vi "Replace Missing Denpendency VIs - Custom gRPC Service Core.vi"(8 "error in":errorcluster, 10 "gRPC Service Name":string, 11 "VI Refnum":refnum<vi>) -> (0 "error out":errorcluster)   [LabVIEW 2023, in "Plugin Generator.lvlib"]
uses:
  Plugin Generator.lvlib
  <vilib>/Utility/traverseref.llb/TRef TravTarget.ctl
  <vilib>/Utility/traverseref.llb/VI Scripting - Traverse.lvlib
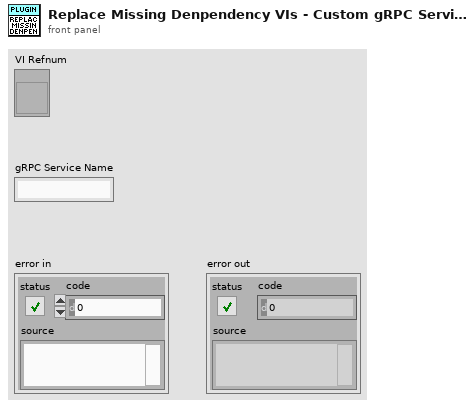
[diagram p1: front panel]
types:
  T1 = typedef "TRef TravTarget.ctl" = enum16{"FP", "BD", "Other"}
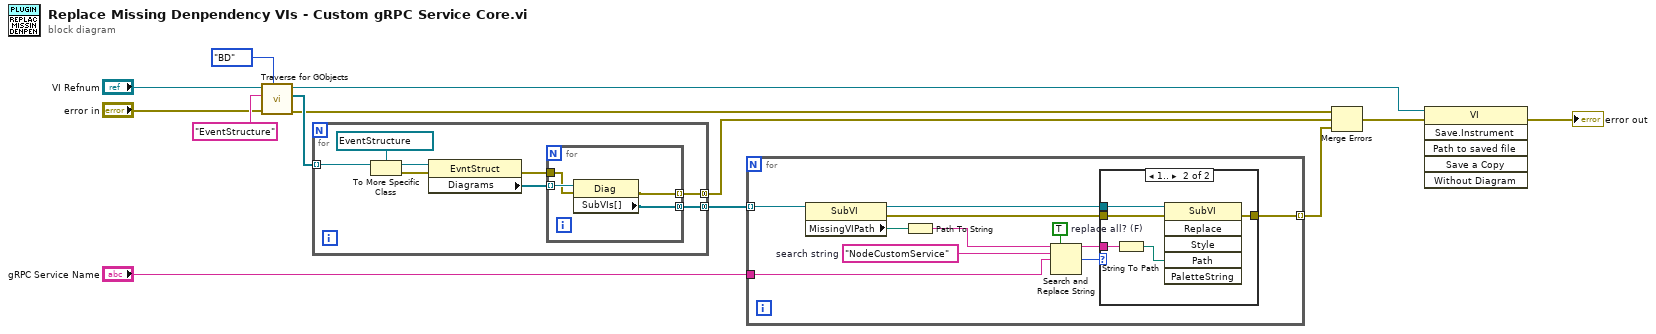
[diagram p0: block diagram]
diagram:
  n1 = call <vilib>:"Traverse for GObjects.vi"("Traverse Target"=TRef_TravTarget."BD", "error in (no error)"="error in", "Class Name"="EventStructure", "VI Refnum"="VI Refnum") -> ("error out"=w4:errorcluster, "References"=w10:refnum<vi>[], "dup VI Refnum"=w11:refnum<vi>)  [unwired: 4 in, 1 out]
  n2 = for {
    tunnel: w10 -> [w21] mode=indexing
    tunnel: [w18] -> w9 mode=concatenating
    tunnel: [w14] -> w3 mode=concatenating
    n3 = To More Specific Class(target class=refnum<vi> refnum ("x"), reference=w21) -> (specific class reference=w20:refnum<vi>, error out=w16:errorcluster)  [unwired: 1 in]
    n4 = property class="EvntStruct"(reference=w20, error in=w16) -> (error out=w15:errorcluster, "Diagrams"=w19:refnum<vi>[])  [unwired: 1 out]
    n5 = for {
      tunnel: w19 -> [w25] mode=indexing
      tunnel: [w24] -> w18 mode=concatenating
      tunnel: w15 -> [w23]
      tunnel: [w22] -> w14 mode=indexing
      n6 = property class="Diag"(reference=w25, error in=w23) -> (error out=w22:errorcluster, "SubVIs[]"=w24:refnum<vi>[])  [unwired: 1 out]
    }
  }
  n7 = for {
    tunnel: w9 -> [w36] mode=indexing
    tunnel: "gRPC Service Name" -> [w34]
    tunnel: [w26] -> w2 mode=indexing
    w30 = TRUE  # replace all? (F)
    w32 = "NodeCustomService"  # search string
    n8 = property class="SubVI"(reference=w36) -> (reference out=w35:refnum<vi>, error out=w27:errorcluster, "MissingVIPath"=w28:path)  [unwired: 1 in]
    n9 = Path To String(path=w28) -> (string=w33:string)
    n10 = Search and Replace String(replace all?=w30, input string=w33, search string=w32, replace string=w34) -> (result string=w31:string, number of replacements=w29:i32)  [unwired: 4 in, 2 out]
    n11 = case shown="1.." w29 {
      tunnel: w35 -> [_ w42]
      tunnel: w31 -> [_ w41]
      tunnel: w27 -> [w37 w39]
      tunnel: [w37 w38] -> w26
      frame Default {
      }
      frame 1.. {
        n12 = String To Path(string=w41) -> (path=w40:path)
        n13 = invoke class="SubVI" method="Replace"(reference=w42, error in=w39, "Path"=w40) -> (error out=w38:errorcluster)  [unwired: 3 in, 5 out]
      }
    }
  }
  n14 = Merge Errors(w4, w3, w2) -> (w5:errorcluster)
  n15 = invoke class="VI" method="Save.Instrument"(reference=w11, error in=w5) -> (error out=→"error out":errorcluster)  [unwired: 4 in, 5 out]
